vi "Create.vi"(8 "error in (no error)":errorcluster, 10 "Parent Name":string) -> (0 "error out":errorcluster, 3 "Redlines Module out":refnum<class "Redlines Module.lvclass">)   [LabVIEW 2020, in "VolatusData.lvlib" / "Redlines Module.lvclass"]
uses:
  Redlines Module.lvclass
  Redlines Module.lvclass/Redlines Module.ctl
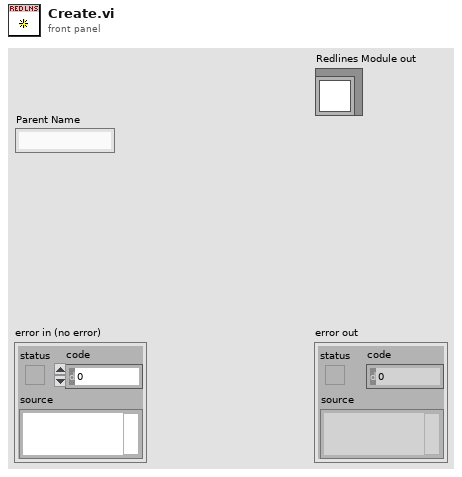
[diagram p1: front panel]
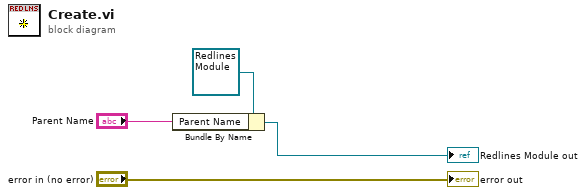
[diagram p0: block diagram]
diagram:
  n1 = Bundle By Name(cluster=refnum<class "Redlines Module.lvclass"> refnum ("Redlines Module in"), "Parent Name"="Parent Name") -> (→"Redlines Module out":refnum<class "Redlines Module.lvclass">)
  "error out" <- "error in (no error)"
